vi "Obtain.vi"(7 "Max Size (-1=Unlimited)":i32=-1, 8 "error in (no error)":errorcluster, 9 "Create if not Found? (T)":bool=TRUE, 11 "Queue Name (\"\"=Unnamed)":string) -> (0 "error out":errorcluster, 1 "Created New?":bool, 3 "Queue out":refnum<queue>)   [LabVIEW 2018, in "Queue.lvlib"]
uses:
  Queue.lvlib
  <vilib>/ErrorRing/Error Ring.xnode
  <vilib>/Utility/error.llb/Error Cluster From Error Code.vi
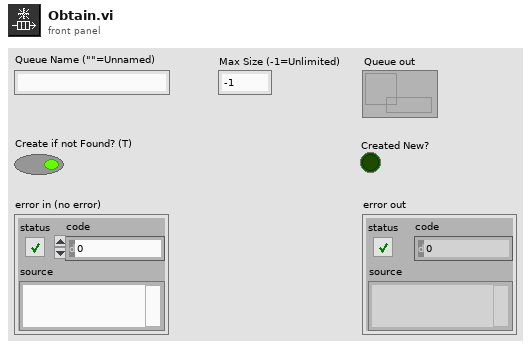
[diagram p1: front panel]
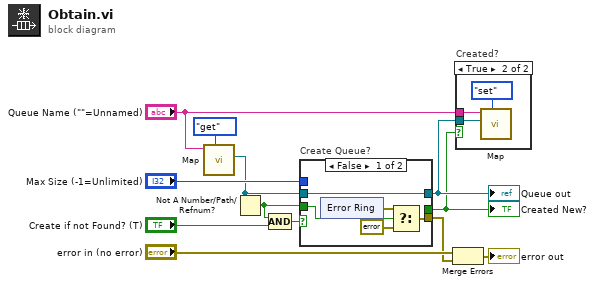
[diagram p0: block diagram]
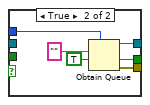
[diagram p3: hidden frame]
diagram:
  n1 = call "Map.vi"("Action"=enum8{"noop", "get", "set", "pop"}."get", "Queue Name"="Queue Name (\"\"=Unnamed)") -> ("Queue out"=w4:refnum<queue>)  [unwired: 8 in, 1 out]
  n2 = Not A Number/Path/Refnum?(number/path/refnum=w4) -> (NaN/Path/Refnum?=w6:bool)
  n3 = Compound Arithmetic op=AND(w6, "Create if not Found? (T)") -> (w7:bool)
  n4 = case "Create Queue?" shown="False" w7 {
    tunnel: "Max Size (-1=Unlimited)" -> [_ w27]
    tunnel: [w17 w26] -> w2
    tunnel: [w16 w25] -> w9
    tunnel: [_ w24] -> w1
    tunnel: w6 -> [w14 _]
    tunnel: w4 -> [w17 _]
    frame False {
      n5 = xnode "Error Ring"() -> ("error out"=w15:errorcluster)
      n6 = Select(t=w15, s=w14, f=errorcluster {"status"=FALSE, "code"=0, "source"=""}) -> (s? t:f=w16:errorcluster)
    }
    frame True {
      n7 = Obtain Queue(max queue size (-1, unlimited)=w27, element data type="", create if not found? (T)=TRUE) -> (queue out=w26:refnum<queue>, created new?=w24:bool, error out=w25:errorcluster)  [unwired: 2 in]
    }
  }
  "Queue out" <- w2
  "Created New?" <- w1
  n8 = Merge Errors("error in (no error)", w9) -> (→"error out":errorcluster)
  n9 = case "Created?" shown="True" w1 {
    tunnel: "Queue Name (\"\"=Unnamed)" -> [_ w29]
    tunnel: w2 -> [_ w28]
    frame False {
    }
    frame True {
      n10 = call "Map.vi"("Action"=enum8{"noop", "get", "set", "pop"}."set", "Queue in"=w28, "Queue Name"=w29) -> ()  [unwired: 7 in, 2 out]
    }
  }
